vi "retrieveAPI details.vi"() -> ()   [LabVIEW 2020]
panel:
  in  "scan folders":bool
  out "# of elements":i32
  out "error out":errorcluster
  in  "destination file":path
  in  "AIM folder":path
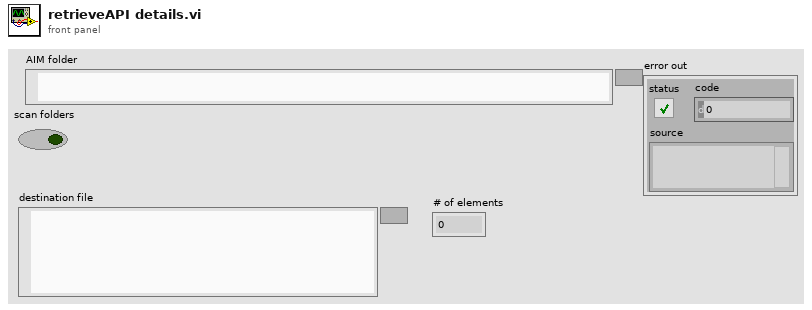
[diagram p1: front panel]
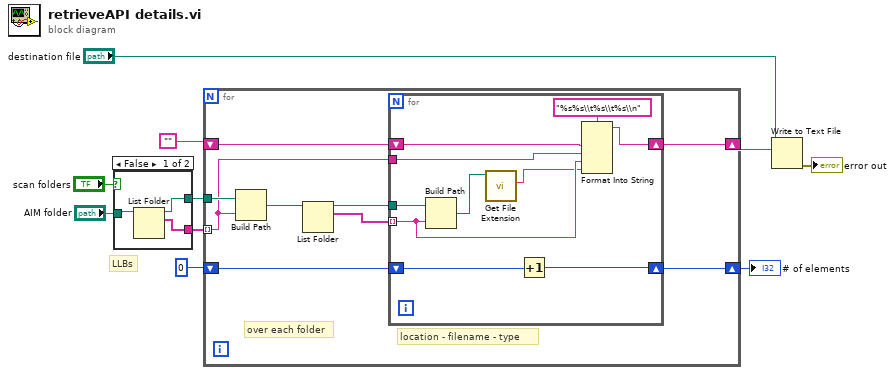
[diagram p0: block diagram]
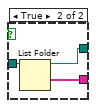
[diagram p2: hidden frame]
diagram:
  # "LLBs"
  n1 = case shown="False" "scan folders" {
    tunnel: "AIM folder" -> [w13 w16]
    tunnel: [w12 w15] -> w9
    tunnel: [w11 w14] -> w2
    frame False {
      n2 = List Folder(path=w13) -> (path out=w12:path, filenames=w11:string[])  [unwired: 3 in, 2 out]
    }
    frame True {
      n3 = List Folder(path=w16) -> (path out=w15:path, folder names=w14:string[])  [unwired: 3 in, 2 out]
    }
  }
  n4 = for {
    tunnel: w2 -> [w20] mode=indexing
    tunnel: w9 -> [w25]
    shift-right: [w19] -> w7
    shift-left: "" -> [w21]
    shift-right: [w17] -> w3
    shift-left: 0 -> [w18]
    # "over each folder"
    # "location - filename - type"
    n5 = Build Path(base path=w25, name or relative path=w20) -> (appended path=w24:path)
    n6 = List Folder(path=w24) -> (path out=w23:path, filenames=w22:string[])  [unwired: 3 in, 2 out]
    n7 = for {
      tunnel: w23 -> [w35]
      tunnel: w22 -> [w27] mode=indexing
      shift-right: [w32] -> w19
      shift-left: w21 -> [w29]
      tunnel: w20 -> [w28]
      shift-right: [w30] -> w17
      shift-left: w18 -> [w31]
      n8 = Build Path(base path=w35, name or relative path=w27) -> (appended path=w34:path)
      n9 = call <vilib>:"Get File Extension.vi"("file"=w34) -> ("lowercase file extension"=w26:string)  [unwired: 6 in, 4 out]
      n10 = Increment(x=w31) -> (x+1=w30:i32)
      n11 = Format Into String(format string="%s%s\\t%s\\t%s\\n", w29, w28, w27, w26) -> (resulting string=w32:string)  [unwired: 2 in, 1 out]
    }
  }
  "# of elements" <- w3
  n12 = Write to Text File(file (use dialog)="destination file", text=w7) -> (error out=→"error out":errorcluster)  [unwired: 2 in, 2 out]
